vi "Logout.vi"(8 "error in (no error)":errorcluster, 11 "Processing in":refnum<class "Processing.lvclass">) -> (0 "error out":errorcluster, 3 "Processing out":refnum<class "Processing.lvclass">)   [LabVIEW 2020, in "HTTP Server.lvlib" / "Processing.lvclass"]
uses:
  Processing.lvclass
  Security/Security.lvclass
  C:/dev/lv20CE/relink/lv-http-server/HTTP Server/Service/Service.lvclass
  Processing.lvclass/Processing.ctl
  Values/Values.lvclass
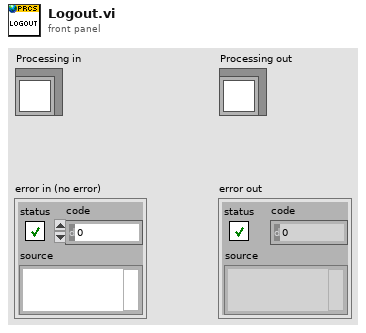
[diagram p1: front panel]
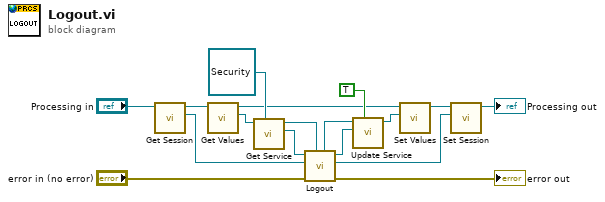
[diagram p0: block diagram]
diagram:
  n1 = call "Get Session.vi"("Processing in"="Processing in") -> ("Session"=w10:refnum<class "Session.lvclass">, "Processing out"=w9:refnum<class "Processing.lvclass">)  [unwired: 9 in]
  n2 = call "Get Values.vi"("Processing in"=w9) -> ("Values"=w17:refnum<class "Values.lvclass">, "Processing out"=w14:refnum<class "Processing.lvclass">)  [unwired: 9 in]
  n3 = call "Get Service.vi"("Service Type"=refnum<class "Security.lvclass"> refnum ("Security in"), "Values in"=w17) -> ("Service"=w12:refnum<class "Security.lvclass">, "Values out"=w7:refnum<class "Values.lvclass">)  [unwired: 7 in, 1 out]
  n4 = call "Logout.vi"("Values In"=w7, "error in (no error)"="error in (no error)", "Session In"=w10, "Security in"=w12) -> ("error out"=→"error out":errorcluster, "Session"=w2:refnum<class "Session.lvclass">, "Security out"=w5:refnum<class "Security.lvclass">, "Values"=w6:refnum<class "Values.lvclass">)  [unwired: 4 in]
  n5 = call "Update Service.vi"("Overwrite? (F)"=TRUE, "Service"=w5, "Values in"=w6) -> ("Values out"=w13:refnum<class "Values.lvclass">)  [unwired: 7 in, 1 out]
  n6 = call "Set Values.vi"("Values"=w13, "Processing in"=w14) -> ("Processing out"=w3:refnum<class "Processing.lvclass">)  [unwired: 9 in]
  n7 = call "Set Session.vi"("Session"=w2, "Processing in"=w3) -> ("Processing out"=→"Processing out":refnum<class "Processing.lvclass">)  [unwired: 9 in]
